vi "set Free Running.vi"(10 "Free Running":bool, 11 "Clock Generator in":refnum<class "Clock Generator.lvclass">) -> (3 "Clock Generator out":refnum<class "Clock Generator.lvclass">)   [LabVIEW 2021, in "Clock Generator.lvclass"]
uses:
  Clock Generator.lvclass
  Clock Generator.lvclass/Clock Generator.ctl
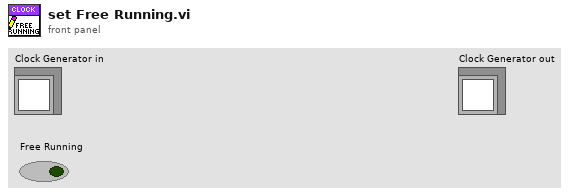
[diagram p1: front panel]
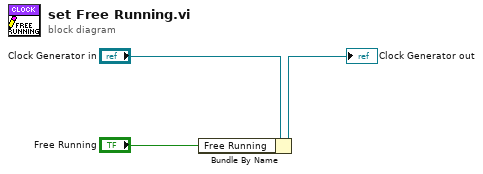
[diagram p0: block diagram]
diagram:
  n1 = Bundle By Name(cluster="Clock Generator in", "Free Running"="Free Running") -> (→"Clock Generator out":refnum<class "Clock Generator.lvclass">)
